vi "Interpolation Scalable.vi"(8 "input valid":bool=TRUE, 9 "x[n].ResampleInfo":T1, 10 "x[n]":fxp<+/-,16,1> format="%.16g", 11 "x[n-1]":fxp<+/-,16,1> format="%.16g") -> (0 "Output Valid":bool, 3 "y[n]":fxp<+/-,22,1> format="%.22g")   [LabVIEW 2010]
uses:
  Controls/ResampleVectorInfo (Single Point).ctl
  <vilib>/rvi/FXPMathLib/basic elements/FxpDiscreteDelay/XNode/nifxpmath_DiscreteDelay.xnode
  <vilib>/rvi/FXPMathLib/FxpSub/XNode/nifxpmath_Sub.xnode
  <vilib>/rvi/FXPMathLib/FxpSub/subVIs/nifxpmath_Sub_SimConfig.ctl
  <vilib>/fxp/LVFixedPointQuantizationPolicyTypeDef.ctl
  <vilib>/fxp/LVFixedPointOverflowPolicyTypeDef.ctl
  <vilib>/rvi/FXPMathLib/FxpMul/XNode/nifxpmath_Multiplier.xnode
  <vilib>/rvi/FXPMathLib/FxpMul/subVIs/nifxpmath_Mul_SimConfig.ctl
  <vilib>/rvi/FXPMathLib/FxpAdd/XNode/nifxpmath_Add.xnode
  <vilib>/rvi/FXPMathLib/FxpAdd/subVIs/nifxpmath_Add_SimConfig.ctl
  <vilib>/rvi/FXPMathLib/FxpSub/simVIs/DllFxpSubTemp_sub.vi
  <vilib>/rvi/FXPMathLib/FxpMul/simVIs/DllFxpMulTemp_sub.vi
  <vilib>/rvi/FXPMathLib/FxpAdd/simVIs/DllFxpAddTemp_sub.vi
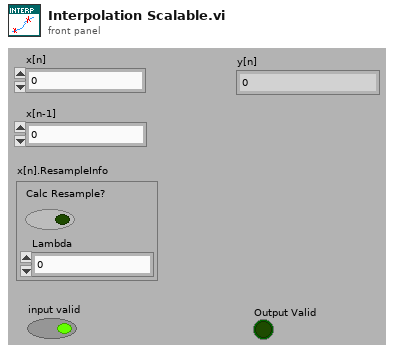
[diagram p1: front panel]
types:
  T1 = typedef "ResampleVectorInfo (Single Point).ctl" = cluster{"Calc Resample?":bool, "Lambda":fxp<+/-,18,1>}
  T2 = cluster{"Calc Resample?":bool, "Lambda":fxp<+/-,18,1>}
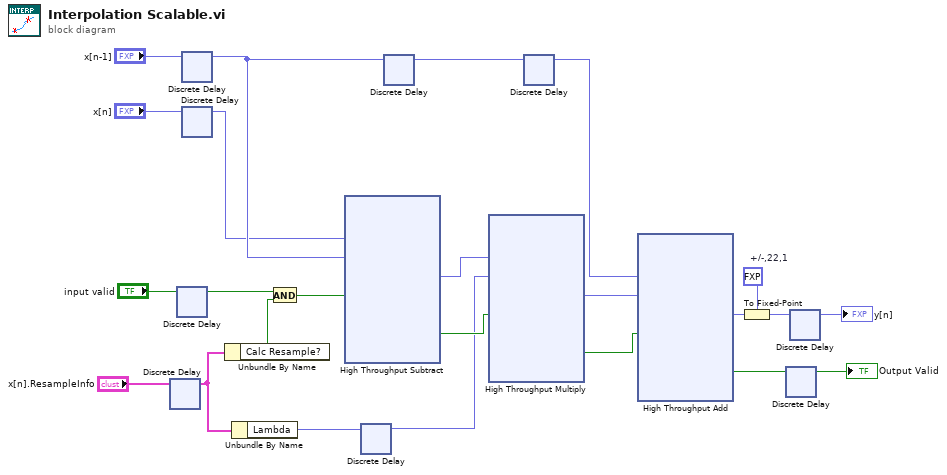
[diagram p0: block diagram]
diagram:
  w9 = fxp<+/-,22,1> 0.0  # +/-,22,1
  n1 = xnode "Discrete Delay"("D"="x[n].ResampleInfo") -> ("Q"=w7:T2)
  n2 = xnode "Discrete Delay"("D"="input valid") -> ("Q"=w5:bool)
  n3 = xnode "Discrete Delay"("D"="x[n-1]") -> ("Q"=w16:fxp<+/-,16,1>)
  n4 = xnode "Discrete Delay"("D"="x[n]") -> ("Q"=w15:fxp<+/-,16,1>)
  n5 = Unbundle By Name(w7) -> ("Calc Resample?"=w6:bool)
  n6 = Unbundle By Name(w7) -> ("Lambda"=w3:fxp<+/-,18,1>)
  n7 = And(x=w5, y=w6) -> (x .and. y?=w4:bool)
  n8 = xnode "High Throughput Subtract"("x"=w15, "y"=w16, "input valid"=w4) -> ("x-y"=w2:fxp<+/-,17,2>, "output valid"=w23:bool)  [unwired: 1 in, 1 out]
  n9 = xnode "Discrete Delay"("D"=w3) -> ("Q"=w1:fxp<+/-,18,1>)
  n10 = xnode "Discrete Delay"("D"=w16) -> ("Q"=w19:fxp<+/-,16,1>)
  n11 = xnode "High Throughput Multiply"("x"=w2, "y"=w1, "input valid"=w23) -> ("x*y"=w10:fxp<+/-,23,2>, "output valid"=w20:bool)  [unwired: 1 in, 1 out]
  n12 = xnode "Discrete Delay"("D"=w19) -> ("Q"=w14:fxp<+/-,16,1>)
  n13 = xnode "High Throughput Add"("x"=w14, "y"=w10, "input valid"=w20) -> ("x+y"=w22:fxp<+/-,24,3>, "output valid"=w12:bool)  [unwired: 1 in, 1 out]
  n14 = To Fixed-Point(fixed-point type=w9, number=w22) -> (fixed-point=w21:fxp<+/-,22,1>)
  n15 = xnode "Discrete Delay"("D"=w12) -> ("Q"=→"Output Valid":bool)
  n16 = xnode "Discrete Delay"("D"=w21) -> ("Q"=→"y[n]":fxp<+/-,22,1>)
